vi "SendMessageDirect.vi"(8 "error in (no error)":errorcluster, 10 "data in":string, 11 "STOMP in":refnum<class "STOMP.lvclass">) -> (0 "error out":errorcluster, 3 "STOMP out":refnum<class "STOMP.lvclass">)   [LabVIEW 2017, in "LabVIEW STOMP.lvlib" / "STOMP.lvclass"]
uses:
  STOMP.lvclass
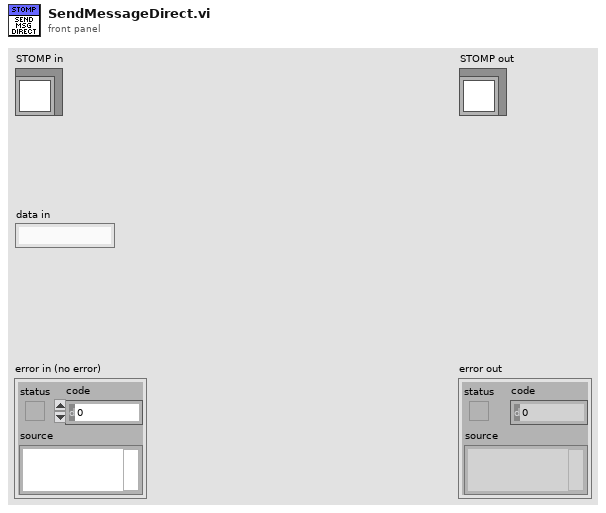
[diagram p1: front panel]
types:
  T1 = typedef "STOMP Connection Manager.lvclass/ObjectAttributes.ctl" = cluster{"address":string, "port":u16, "ConnectionRef":refnum<k5>, "messageQueue":refnum<queue>, "receiptQueue":refnum<queue>, "errorQueue":refnum<queue>, "sendQueue":refnum<queue>, "currentReceiptNumber":u64, "currentSubscriptionId":u64, "closeConnection":bool, "activeSubscriptions":T2[]}
  T2 = typedef "LabVIEW STOMP.lvlib/STOMP.lvclass/Type_ActiveSubscription.ctl" = cluster{"id":u64, "receipt":bool, "Destination":string, "ack":T3, "headers":T4[]}
  T3 = typedef "LabVIEW STOMP.lvlib/STOMP.lvclass/Type_AckHeader.ctl" = enum16{"auto", "client", "client-individual"}
  T4 = typedef "LabVIEW STOMP.lvlib/STOMP.lvclass/Type_FrameHeader.ctl" = cluster{"Header":string, "Value":string}
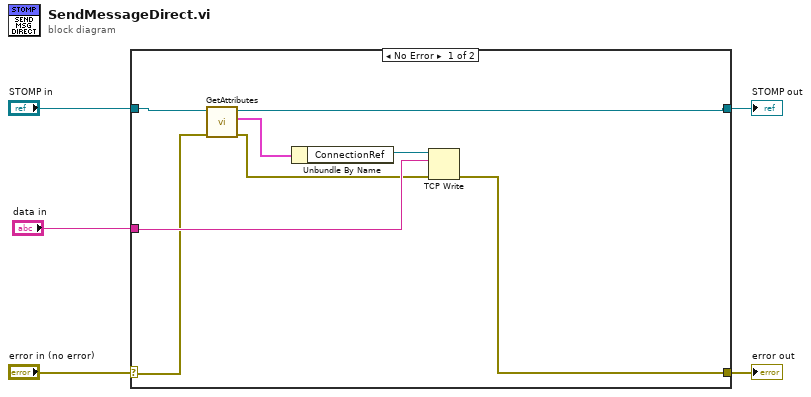
[diagram p0: block diagram]
diagram:
  n1 = case shown="No Error" "error in (no error)" {
    selector: "error in (no error)" -> [w7 w15]
    tunnel: [w11 w15] -> w4
    tunnel: [w8 w14] -> w2
    tunnel: "STOMP in" -> [w10 w14]
    tunnel: "data in" -> [w12 _]
    frame No Error {
      n2 = call-dynamic "GetAttributes.vi"("error in (no error)"=w7, "STOMP in"=w10) -> ("error out"=w6:errorcluster, "attributes"=w9:T1, "STOMP out"=w8:refnum<class "STOMP.lvclass">)  [unwired: 7 in]
      n3 = Unbundle By Name(w9) -> ("ConnectionRef"=w13:refnum<k5>)
      n4 = TCP Write(connection ID=w13, data in=w12, error in (no error)=w6) -> (error out=w11:errorcluster)  [unwired: 1 in, 2 out]
    }
    frame Error {
    }
  }
  "error out" <- w4
  "STOMP out" <- w2
